vi "读写配置文件.vi"(8 "BoardConfig_input":T1, 9 "m_bCreat":bool, 10 "文件名称":string, 11 "m_bRead":bool) -> (2 "BoardConfig_output":T1)   [LabVIEW 2010]
doc: "读写以太网配置文件\n\n参数 m_bRead：\nTRUE 为读配置 FALSE 为写配置\n\n参数 io_put_write：\n当 m_bRead 为 FALSE 写配置时 如果该值为 0 表示写输入配置 1 表示写输出配置"
uses:
  <vilib>/Utility/config.llb/Write Key (I32).vi
  <vilib>/Utility/config.llb/Write Key (U32).vi
  <vilib>/Utility/config.llb/Write Key (Double).vi
  <vilib>/Utility/config.llb/Write Key (Boolean).vi
  <vilib>/Utility/config.llb/Write Key (String).vi
  <vilib>/Utility/config.llb/Read Key (U32).vi
  <vilib>/Utility/config.llb/Read Key (Double).vi
  <vilib>/Utility/config.llb/Read Key (I32).vi
  <vilib>/Utility/config.llb/Read Key (Boolean).vi
  <vilib>/Utility/config.llb/Read Key (String).vi
  <vilib>/Utility/config.llb/NI_LVConfig.lvlib
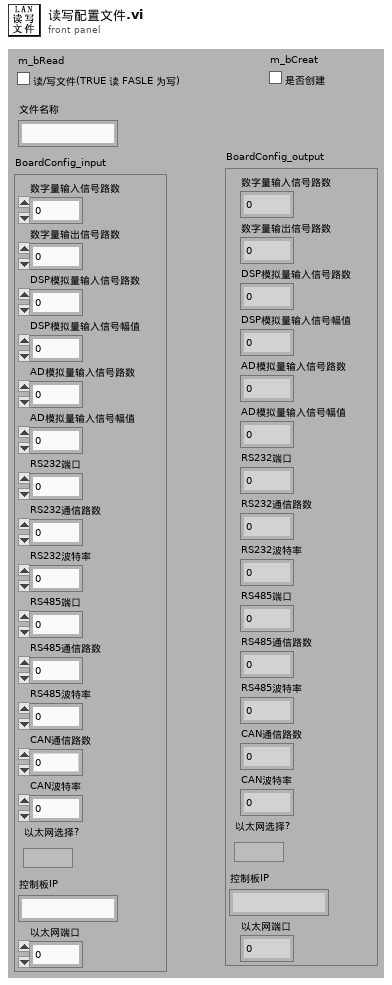
[diagram p1: front panel]
types:
  T1 = cluster{"数字量输入信号路数":i32, "数字量输出信号路数":i32, "DSP模拟量输入信号路数":u32, "DSP模拟量输入信号幅值":u32, "AD模拟量输入信号路数":u32, "AD模拟量输入信号幅值":u32, "RS232端口":u32, "RS232通信路数":u32, "RS232波特率":dbl, "RS485端口":u32, "RS485通信路数":u32, "RS485波特率":u32, "CAN通信路数":i32, "CAN波特率":u32, "以太网选择?":bool, "控制板IP":string, "以太网端口":u32}
  T2 = typedef "NI_LVConfig.lvlib/Config Data RefNum.ctl" = refnum<k1>
  T3 = cluster{"value":u32, "value":u32, "value":u32, "value":u32, "value":u32, "value":u32, "value":u32, "value":u32, "value":dbl, "value":u32, "value":u32, "value":u32, "value":i32, "value":u32, "value":bool, "value":string, "value":u32}
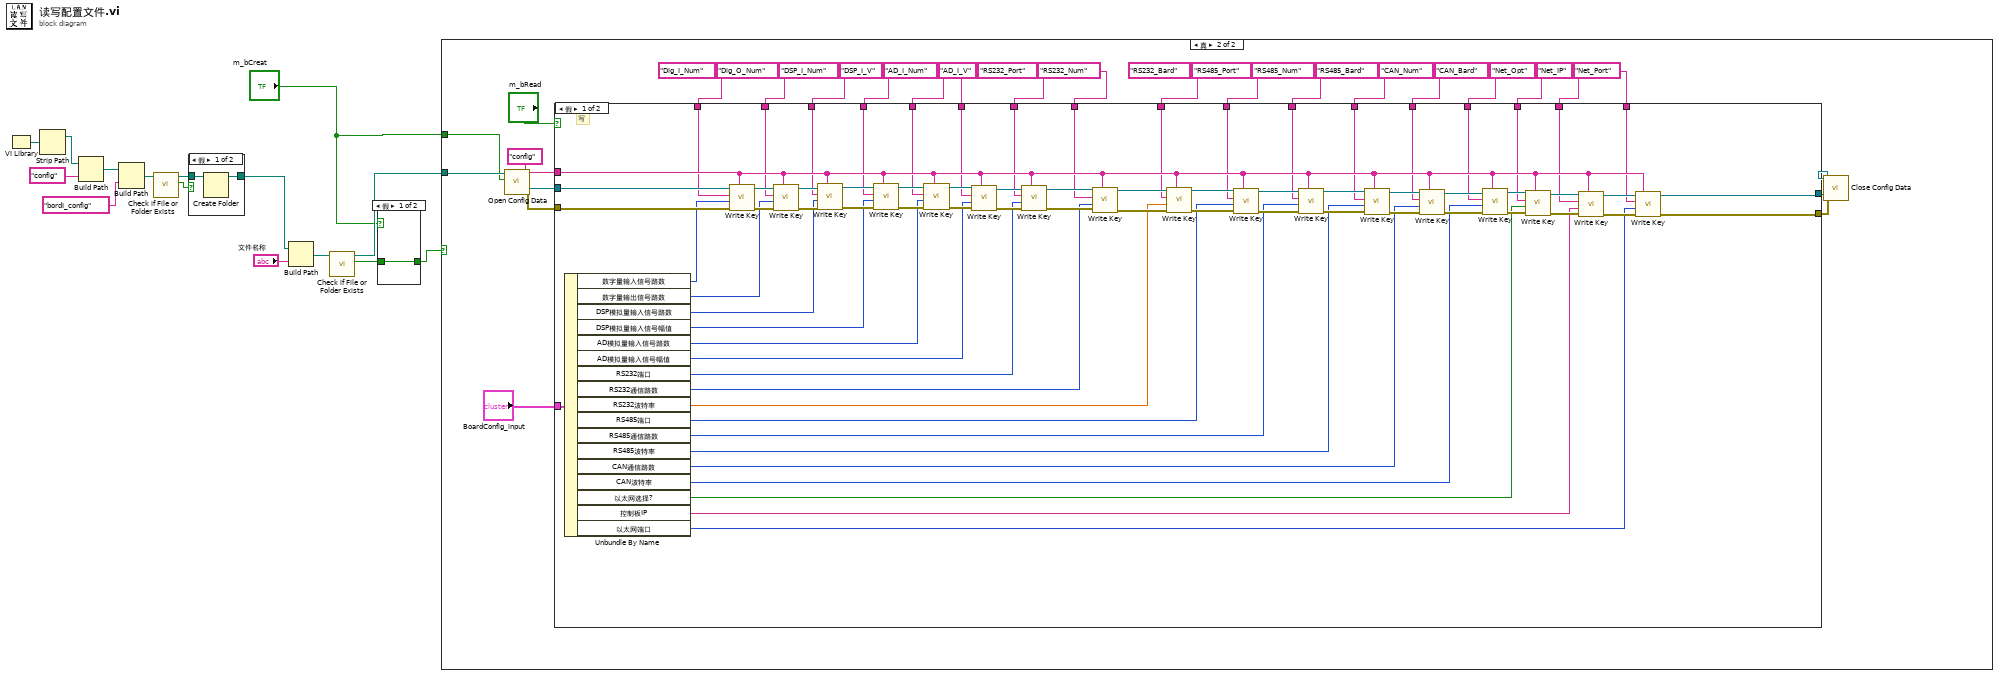
[diagram p0: block diagram]
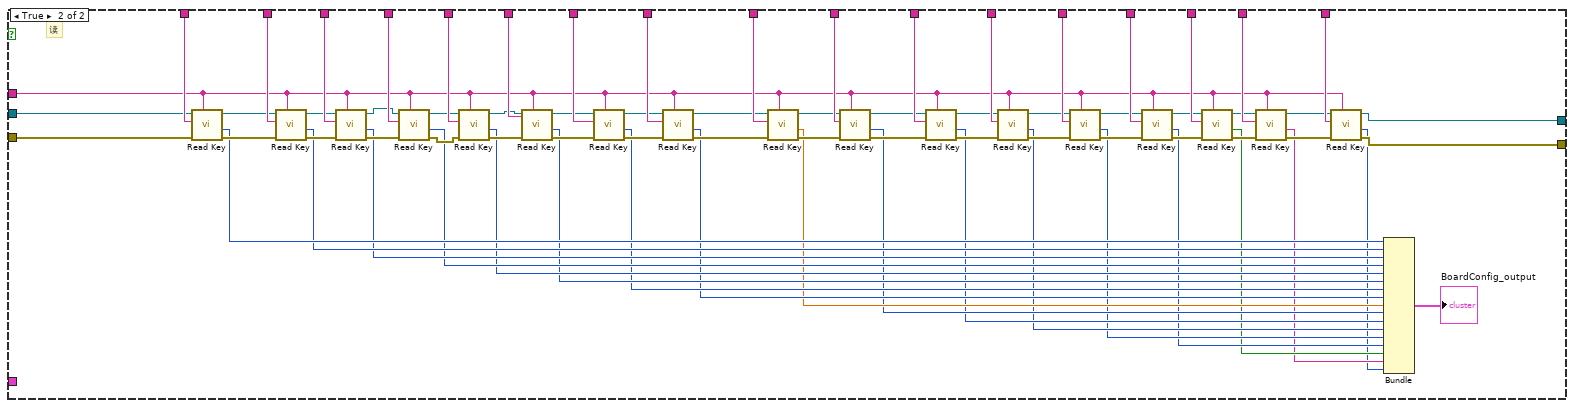
[diagram p3: hidden frame]
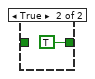
[diagram p4: hidden frame]
diagram:
  n1 = VI Library() -> (path=w14:path)
  n2 = Strip Path(path=w14) -> (stripped path=w15:path)  [unwired: 1 out]
  n3 = Build Path(base path=w15, name or relative path="config") -> (appended path=w8:path)
  n4 = Build Path(base path=w8, name or relative path="bordI_config" ("名称或相对路径")) -> (appended path=w7:path)
  n5 = call <vilib>:"Check if File or Folder Exists.vi"("path"=w7) -> ("file or folder exists?"=w12:bool, "dup path"=w11:path)  [unwired: 8 in, 1 out]
  n6 = case shown="假" w12 {
    tunnel: w11 -> [w16 w18]
    tunnel: [w17 w18] -> w10
    frame False {
      n7 = Create Folder(path (use dialog)=w16) -> (created path=w17:path)  [unwired: 2 in, 2 out]
    }
    frame True {
    }
  }
  n8 = Build Path(base path=w10, name or relative path="文件名称") -> (appended path=w5:path)
  n9 = call <vilib>:"Check if File or Folder Exists.vi"("path"=w5) -> ("file or folder exists?"=w3:bool, "dup path"=w4:path)  [unwired: 8 in, 1 out]
  n10 = case shown="假" "m_bCreat" {
    tunnel: [w19 TRUE] -> w2
    tunnel: w3 -> [w19 _]
    frame False {
    }
    frame True {
    }
  }
  n11 = case shown="真" w2 {
    tunnel: w4 -> [_ w46]
    tunnel: "m_bCreat" -> [_ w21]
    frame False {
    }
    frame True {
      n12 = call <vilib>:"Open Config Data.vi"("create file if necessary (T)"=w21, "configuration file path"=w46) -> ("error out"=w43:errorcluster, "refnum"=w44:T2)  [unwired: 7 in, 1 out]
      n13 = case shown="假" "m_bRead" {
        tunnel: w44 -> [w118 w173]
        tunnel: w43 -> [w117 w172]
        tunnel: "config" -> [w72 w137]
        tunnel: [w74 w149] -> w41
        tunnel: [w73 w138] -> w40
        tunnel: "BoardConfig_input" -> [w114 _]
        tunnel: "Dig_I_Num" ("key") -> [w63 w190]
        tunnel: "Dig_O_Num" ("key") -> [w62 w189]
        tunnel: "DSP_I_Num" ("key") -> [w61 w188]
        tunnel: "DSP_I_V" ("key") -> [w60 w187]
        tunnel: "AD_I_Num" ("key") -> [w59 w186]
        tunnel: "AD_I_V" ("key") -> [w58 w185]
        tunnel: "RS232_Port" ("key") -> [w57 w184]
        tunnel: "RS232_Num" ("key") -> [w56 w183]
        tunnel: "RS232_Bard" ("key") -> [w55 w182]
        tunnel: "RS485_Port" ("key") -> [w54 w181]
        tunnel: "RS485_Num" ("key") -> [w53 w180]
        tunnel: "RS485_Bard" ("key") -> [w52 w179]
        tunnel: "CAN_Num" ("key") -> [w51 w178]
        tunnel: "CAN_Bard" ("key") -> [w50 w177]
        tunnel: "Net_Opt" ("key") -> [w49 w176]
        tunnel: "Net_IP" ("key") -> [w48 w175]
        tunnel: "Net_Port" ("key") -> [w47 w174]
        frame False {
          # "写"
          n14 = Unbundle By Name(w114) -> ("数字量输入信号路数"=w113:i32, "数字量输出信号路数"=w110:i32, "DSP模拟量输入信号路数"=w107:u32, "DSP模拟量输入信号幅值"=w104:u32, "AD模拟量输入信号路数"=w103:u32, "AD模拟量输入信号幅值"=w100:u32, "RS232端口"=w97:u32, "RS232通信路数"=w92:u32, "RS232波特率"=w91:dbl, "RS485端口"=w71:u32, "RS485通信路数"=w70:u32, "RS485波特率"=w69:u32, "CAN通信路数"=w68:i32, "CAN波特率"=w67:u32, "以太网选择?"=w66:bool, "控制板IP"=w65:string, "以太网端口"=w64:u32)
          n15 = call-poly <vilib>:"Write Key.vi"("section"=w72, "error in (no error)"=w117, "value"=w113, "key"=w63, "refnum"=w118) -> ("error out"=w111:errorcluster, "refnum out"=w112:T2)  [unwired: 4 in, 1 out]
          n16 = call-poly <vilib>:"Write Key.vi"("section"=w72, "error in (no error)"=w111, "value"=w110, "key"=w62, "refnum"=w112) -> ("error out"=w108:errorcluster, "refnum out"=w109:T2)  [unwired: 4 in, 1 out]
          n17 = call-poly <vilib>:"Write Key.vi"("section"=w72, "error in (no error)"=w108, "value"=w107, "key"=w61, "refnum"=w109) -> ("error out"=w105:errorcluster, "refnum out"=w106:T2)  [unwired: 4 in, 1 out]
          n18 = call-poly <vilib>:"Write Key.vi"("section"=w72, "error in (no error)"=w105, "value"=w104, "key"=w60, "refnum"=w106) -> ("error out"=w115:errorcluster, "refnum out"=w116:T2)  [unwired: 4 in, 1 out]
          n19 = call-poly <vilib>:"Write Key.vi"("section"=w72, "error in (no error)"=w115, "value"=w103, "key"=w59, "refnum"=w116) -> ("error out"=w101:errorcluster, "refnum out"=w102:T2)  [unwired: 4 in, 1 out]
          n20 = call-poly <vilib>:"Write Key.vi"("section"=w72, "error in (no error)"=w101, "value"=w100, "key"=w58, "refnum"=w102) -> ("error out"=w99:errorcluster, "refnum out"=w98:T2)  [unwired: 4 in, 1 out]
          n21 = call-poly <vilib>:"Write Key.vi"("section"=w72, "error in (no error)"=w99, "value"=w97, "key"=w57, "refnum"=w98) -> ("error out"=w96:errorcluster, "refnum out"=w95:T2)  [unwired: 4 in, 1 out]
          n22 = call-poly <vilib>:"Write Key.vi"("section"=w72, "error in (no error)"=w96, "value"=w92, "key"=w56, "refnum"=w95) -> ("error out"=w93:errorcluster, "refnum out"=w94:T2)  [unwired: 4 in, 1 out]
          n23 = call-poly <vilib>:"Write Key.vi"("section"=w72, "error in (no error)"=w93, "value"=w91, "key"=w55, "refnum"=w94) -> ("error out"=w86:errorcluster, "refnum out"=w87:T2)  [unwired: 4 in, 1 out]
          n24 = call-poly <vilib>:"Write Key.vi"("section"=w72, "error in (no error)"=w86, "value"=w71, "key"=w54, "refnum"=w87) -> ("error out"=w85:errorcluster, "refnum out"=w88:T2)  [unwired: 4 in, 1 out]
          n25 = call-poly <vilib>:"Write Key.vi"("section"=w72, "error in (no error)"=w85, "value"=w70, "key"=w53, "refnum"=w88) -> ("error out"=w83:errorcluster, "refnum out"=w84:T2)  [unwired: 4 in, 1 out]
          n26 = call-poly <vilib>:"Write Key.vi"("section"=w72, "error in (no error)"=w83, "value"=w69, "key"=w52, "refnum"=w84) -> ("error out"=w81:errorcluster, "refnum out"=w82:T2)  [unwired: 4 in, 1 out]
          n27 = call-poly <vilib>:"Write Key.vi"("section"=w72, "error in (no error)"=w81, "value"=w68, "key"=w51, "refnum"=w82) -> ("error out"=w89:errorcluster, "refnum out"=w90:T2)  [unwired: 4 in, 1 out]
          n28 = call-poly <vilib>:"Write Key.vi"("section"=w72, "error in (no error)"=w89, "value"=w67, "key"=w50, "refnum"=w90) -> ("error out"=w79:errorcluster, "refnum out"=w80:T2)  [unwired: 4 in, 1 out]
          n29 = call-poly <vilib>:"Write Key.vi"("section"=w72, "error in (no error)"=w79, "value"=w66, "key"=w49, "refnum"=w80) -> ("error out"=w77:errorcluster, "refnum out"=w78:T2)  [unwired: 4 in, 1 out]
          n30 = call-poly <vilib>:"Write Key.vi"("section"=w72, "error in (no error)"=w77, "value"=w65, "key"=w48, "refnum"=w78) -> ("error out"=w75:errorcluster, "refnum out"=w76:T2)  [unwired: 4 in, 1 out]
          n31 = call-poly <vilib>:"Write Key.vi"("section"=w72, "error in (no error)"=w75, "value"=w64, "key"=w47, "refnum"=w76) -> ("error out"=w73:errorcluster, "refnum out"=w74:T2)  [unwired: 4 in, 1 out]
        }
        frame True {
          # "读"
          n32 = call-poly <vilib>:"Read Key.vi"("section"=w137, "error in (no error)"=w172, "key"=w190, "refnum"=w173) -> ("error out"=w170:errorcluster, "value"=w136:u32, "refnum out"=w171:T2)  [unwired: 4 in, 1 out]
          n33 = call-poly <vilib>:"Read Key.vi"("section"=w137, "error in (no error)"=w170, "key"=w189, "refnum"=w171) -> ("error out"=w168:errorcluster, "value"=w135:u32, "refnum out"=w169:T2)  [unwired: 4 in, 1 out]
          n34 = call-poly <vilib>:"Read Key.vi"("section"=w137, "error in (no error)"=w168, "key"=w188, "refnum"=w169) -> ("error out"=w166:errorcluster, "value"=w134:u32, "refnum out"=w167:T2)  [unwired: 4 in, 1 out]
          n35 = call-poly <vilib>:"Read Key.vi"("section"=w137, "error in (no error)"=w166, "key"=w187, "refnum"=w167) -> ("error out"=w164:errorcluster, "value"=w133:u32, "refnum out"=w165:T2)  [unwired: 4 in, 1 out]
          n36 = call-poly <vilib>:"Read Key.vi"("section"=w137, "error in (no error)"=w164, "key"=w186, "refnum"=w165) -> ("error out"=w162:errorcluster, "value"=w132:u32, "refnum out"=w163:T2)  [unwired: 4 in, 1 out]
          n37 = call-poly <vilib>:"Read Key.vi"("section"=w137, "error in (no error)"=w162, "key"=w185, "refnum"=w163) -> ("error out"=w160:errorcluster, "value"=w131:u32, "refnum out"=w161:T2)  [unwired: 4 in, 1 out]
          n38 = call-poly <vilib>:"Read Key.vi"("section"=w137, "error in (no error)"=w160, "key"=w184, "refnum"=w161) -> ("error out"=w148:errorcluster, "value"=w130:u32, "refnum out"=w159:T2)  [unwired: 4 in, 1 out]
          n39 = call-poly <vilib>:"Read Key.vi"("section"=w137, "error in (no error)"=w148, "key"=w183, "refnum"=w159) -> ("error out"=w147:errorcluster, "value"=w129:u32, "refnum out"=w158:T2)  [unwired: 4 in, 1 out]
          n40 = call-poly <vilib>:"Read Key.vi"("section"=w137, "error in (no error)"=w147, "key"=w182, "refnum"=w158) -> ("error out"=w146:errorcluster, "value"=w128:dbl, "refnum out"=w157:T2)  [unwired: 4 in, 1 out]
          n41 = call-poly <vilib>:"Read Key.vi"("section"=w137, "error in (no error)"=w146, "key"=w181, "refnum"=w157) -> ("error out"=w145:errorcluster, "value"=w127:u32, "refnum out"=w156:T2)  [unwired: 4 in, 1 out]
          n42 = call-poly <vilib>:"Read Key.vi"("section"=w137, "error in (no error)"=w145, "key"=w180, "refnum"=w156) -> ("error out"=w144:errorcluster, "value"=w126:u32, "refnum out"=w155:T2)  [unwired: 4 in, 1 out]
          n43 = call-poly <vilib>:"Read Key.vi"("section"=w137, "error in (no error)"=w144, "key"=w179, "refnum"=w155) -> ("error out"=w143:errorcluster, "value"=w125:u32, "refnum out"=w154:T2)  [unwired: 4 in, 1 out]
          n44 = call-poly <vilib>:"Read Key.vi"("section"=w137, "error in (no error)"=w143, "key"=w178, "refnum"=w154) -> ("error out"=w142:errorcluster, "value"=w124:i32, "refnum out"=w153:T2)  [unwired: 4 in, 1 out]
          n45 = call-poly <vilib>:"Read Key.vi"("section"=w137, "error in (no error)"=w142, "key"=w177, "refnum"=w153) -> ("error out"=w141:errorcluster, "value"=w123:u32, "refnum out"=w152:T2)  [unwired: 4 in, 1 out]
          n46 = call-poly <vilib>:"Read Key.vi"("section"=w137, "error in (no error)"=w141, "key"=w176, "refnum"=w152) -> ("error out"=w140:errorcluster, "value"=w122:bool, "refnum out"=w151:T2)  [unwired: 4 in, 1 out]
          n47 = call-poly <vilib>:"Read Key.vi"("section"=w137, "error in (no error)"=w140, "key"=w175, "refnum"=w151) -> ("error out"=w139:errorcluster, "value"=w121:string, "refnum out"=w150:T2)  [unwired: 4 in, 1 out]
          n48 = call-poly <vilib>:"Read Key.vi"("section"=w137, "error in (no error)"=w139, "key"=w174, "refnum"=w150) -> ("error out"=w138:errorcluster, "value"=w120:u32, "refnum out"=w149:T2)  [unwired: 4 in, 1 out]
          n49 = Bundle("value"=w136, "value"=w135, "value"=w134, "value"=w133, "value"=w132, "value"=w131, "value"=w130, "value"=w129, "value"=w128, "value"=w127, "value"=w126, "value"=w125, "value"=w124, "value"=w123, "value"=w122, "value"=w121, "value"=w120) -> (→"BoardConfig_output":T3)  [unwired: 1 in]
        }
      }
      n50 = call <vilib>:"Close Config Data.vi"("error in (no error)"=w40, "refnum"=w41) -> ()  [unwired: 8 in, 2 out]
    }
  }
